vi "Timer FGV.vi"(9 "Target Time (s)":dbl, 11 "Timer Command":T1) -> (1 "Elapsed Time":dbl, 2 "Done?":bool)   [LabVIEW 2012]
doc: "This VI is a functional global variable that keeps track the amount of time elapsed since a Start command was sent to the VI."
uses:
  TimerCommands.ctl
panel:
  # "Input"
  # "Output"
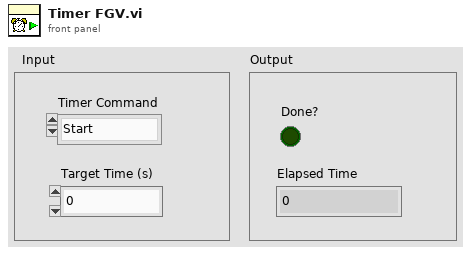
[diagram p1: front panel]
types:
  T1 = typedef "TimerCommands.ctl" = enum16{"Start", "Check Time"}
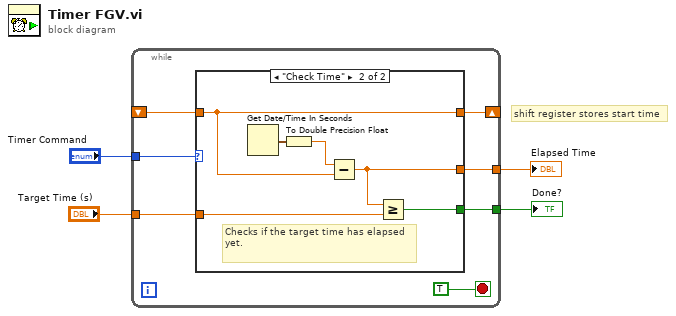
[diagram p0: block diagram]
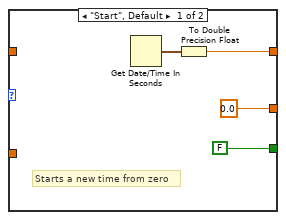
[diagram p2: hidden frame]
diagram:
  # "shift register stores start time"
  n1 = while {
    tunnel: "Timer Command" -> [w11]
    shift-right: [w10] -> _
    shift-left: _ -> [w9]
    tunnel: [w8] -> w3
    tunnel: [w7] -> w2
    tunnel: "Target Time (s)" -> [w6]
    stop <- TRUE stop-if-true
    n2 = case shown="\"Check Time\"" w11 {
      tunnel: [w14 w19] -> w10
      tunnel: w9 -> [_ w19]
      tunnel: [0.0 ("double precision float") w18] -> w8
      tunnel: [FALSE w17] -> w7
      tunnel: w6 -> [_ w16]
      frame "Start", Default {
        # "Starts a new time from zero"
        n3 = Get Date/Time In Seconds() -> (seconds since 1Jan1904=w15:timestamp)
        n4 = To Double Precision Float(number=w15) -> (double precision float=w14:dbl)
      }
      frame "Check Time" {
        # "Checks if the target time has elapsed yet."
        n5 = Get Date/Time In Seconds() -> (seconds since 1Jan1904=w21:timestamp)
        n6 = To Double Precision Float(number=w21) -> (double precision float=w20:dbl)
        n7 = Subtract(x=w20, y=w19) -> (x-y=w18:dbl)
        n8 = Greater Or Equal?(x=w18, y=w16) -> (x >= y?=w17:bool)
      }
    }
  }
  "Elapsed Time" <- w3
  "Done?" <- w2
